vi "formas_cc.vi"(4 "retardo":dbl, 5 "Numerador":dbl[](array[numeric]), 6 "Denominador":dbl[](array[numeric])) -> (0 "Vector C":dbl[](array[numeric]), 1 "Vector B":dbl[](array[numeric]), 2 "Matriz A":T1)   [LabVIEW 2019]
doc: "Transforma una ecuacion del comportamiento del sistema( FT), a su representacion en el espacios de estados , con su numerador ,denominador y un retardo si se tiene , entregando la formas FCO."
uses:
  <vilib>/Analysis/Matrix/Datatypes/RealMatrix.ctl
  <vilib>/Analysis/7linalg.llb/Create Special Real Matrix.vi
  <vilib>/Analysis/NI_AALPro.lvlib
  <vilib>/Analysis/Matrix/NI_Matrix.lvlib
panel:
  out "Numerador 2":dbl[](array[numeric])
  out "Denominador 2":dbl[](array[numeric])
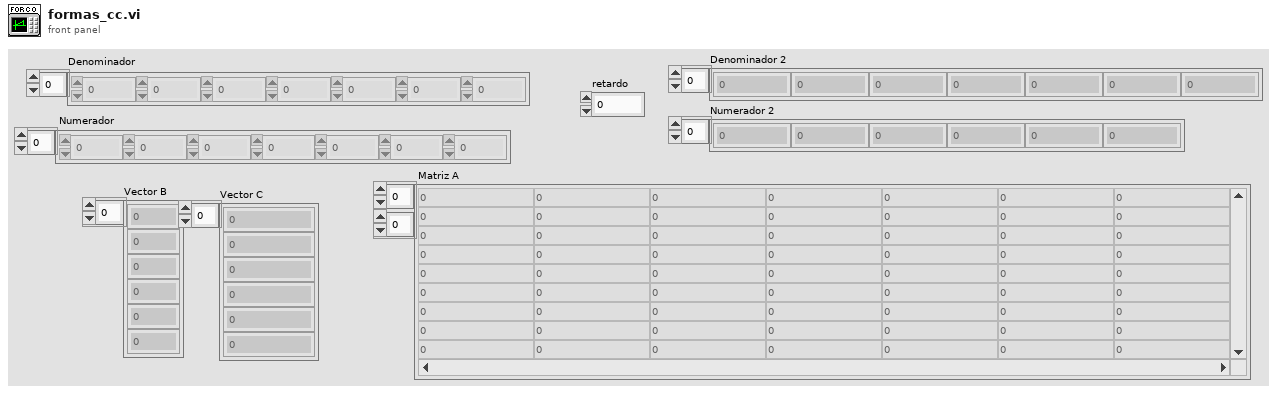
[diagram p1: front panel]
types:
  T1 = typedef "NI_Matrix.lvlib/RealMatrix.ctl" = dbl[][]
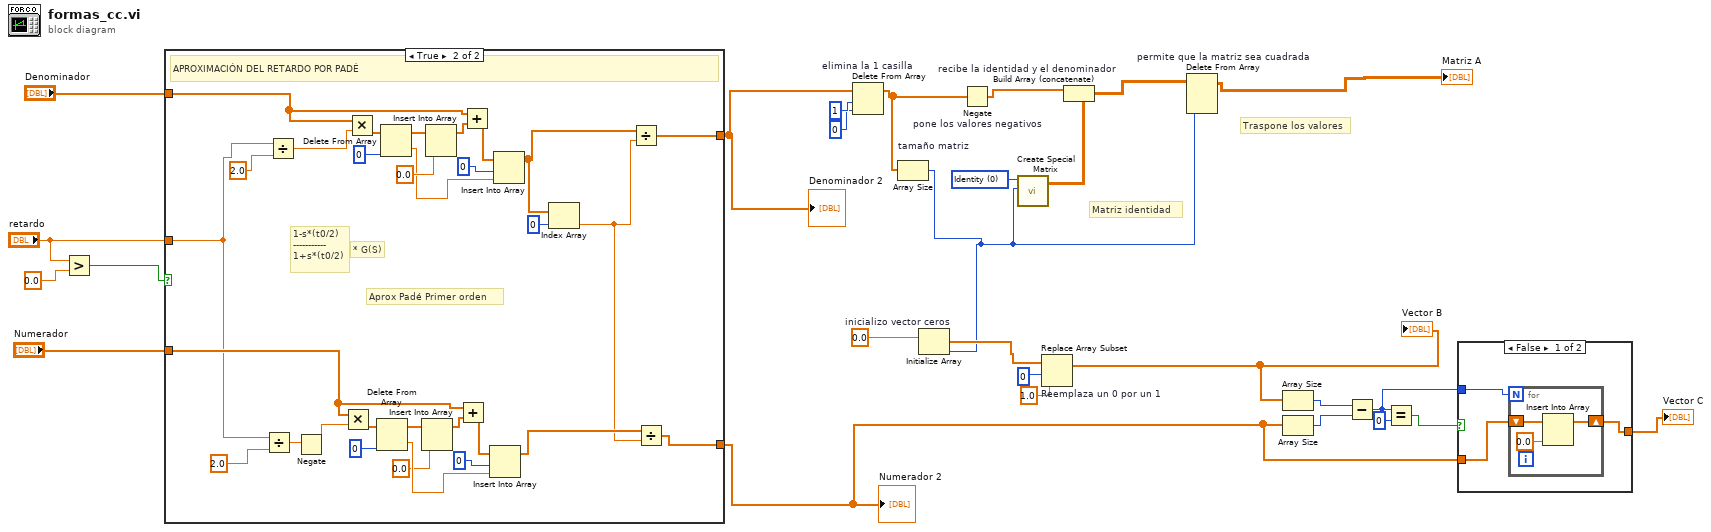
[diagram p0: block diagram]
diagram:
  w21 = 0 items=["Identity", "Diagonal", "Toeplitz", "Vandermonde", "Companion", "Hankel", "Hadamard", "Wilkinson", "Hilbert", "Inverse Hilbert", "Rosser", "Pascal"] ("matrix type")
  # "Matriz identidad"
  # "Traspone los valores"
  n1 = Greater?(x="retardo", y=0.0) -> (0:w11:bool)
  n2 = case shown="True" w11 {
    tunnel: "Numerador" -> [w28 w55]
    tunnel: "retardo" -> [_ w39]
    tunnel: "Denominador" -> [w29 w38]
    tunnel: [w28 w37] -> w3
    tunnel: [w29 w35] -> w9
    frame False {
    }
    frame True {
      # "* G(S)"
      # "Aprox Padé Primer orden"
      # "1-s*(t0/2)\n-----------\n1+s*(t0/2)"
      # "APROXIMACIÓN DEL RETARDO POR PADÉ"
      n3 = Divide(x=w39, y=2.0) -> (x/y=w36:dbl)
      n4 = Divide(x=w39, y=2.0) -> (x/y=w34:dbl)
      n5 = Negate(x=w36) -> (-x=w57:dbl)
      n6 = Multiply(x=w55, y=w57) -> (x*y=w56:dbl[])
      n7 = Multiply(x=w38, y=w34) -> (x*y=w42:dbl[])
      n8 = Delete From Array(array=w56, index=0) -> (deleted portion=w54:dbl, array with subset deleted=w52:dbl[])  [unwired: 1 in]
      n9 = Delete From Array(array=w42, index=0) -> (deleted portion=w43:dbl, array with subset deleted=w45:dbl[])  [unwired: 1 in]
      n10 = Insert Into Array(array=w52, new element=0.0 ("new element/subarray")) -> (w49:dbl[])  [unwired: 1 in]
      n11 = Insert Into Array(array=w45, new element=0.0 ("new element/subarray")) -> (w48:dbl[])  [unwired: 1 in]
      n12 = Add(x=w55, y=w49) -> (x+y=w53:dbl[])
      n13 = Add(x=w38, y=w48) -> (x+y=w44:dbl[])
      n14 = Insert Into Array(array=w53, index=0, new element=w54) -> (w31:dbl[])
      n15 = Insert Into Array(array=w44, index=0, new element=w43) -> (w33:dbl[])
      n16 = Index Array(array=w33, index=0) -> (element=w30:dbl)
      n17 = Divide(x=w33, y=w30) -> (x/y=w35:dbl[])
      n18 = Divide(x=w31, y=w30) -> (x/y=w37:dbl[])
    }
  }
  "Denominador 2" <- w9
  "Numerador 2" <- w3
  n19 = Delete From Array "elimina la 1 casilla"(array=w9, length=1, index=0) -> (array with subset deleted=w23:dbl[])  [unwired: 1 out]
  n20 = Array Size "tamaño matriz"(array=w23) -> (size(s)=w13:i32)
  n21 = Initialize Array "inicializo vector ceros"(0.0 ("element"), w13) -> (w17:dbl[])
  n22 = Negate "pone los valores negativos"(x=w23) -> (-x=w22:dbl[])
  n23 = call-poly <vilib>:"Create Special Matrix.vi"("matrix type"=w21, "matrix size"=w13) -> ("Special Matrix"=w20:T1)  [unwired: 3 in, 1 out]
  n24 = Replace Array Subset "Reemplaza un 0 por un 1"(array=w17, new element=1.0 ("new element/subarray"), index=0) -> (w8:dbl[])
  "Vector B" <- w8
  n25 = Build Array (concatenate) "recibe la identidad y el denominador"(w22, w20) -> (w19:T1)
  n26 = Delete From Array "permite que la matriz sea cuadrada"(array=w19, index (row)=w13) -> (array with subset deleted=→"Matriz A":T1)  [unwired: 2 in, 1 out]
  n27 = Array Size(array=w8) -> (size(s)=w7:i32)
  n28 = Array Size(array=w3) -> (size(s)=w6:i32)
  n29 = Subtract(x=w7, y=w6) -> (x-y=w1:i32)
  n30 = Equal?(x=w1, y=0) -> (x = y?=w4:bool)
  n31 = case shown="False" w4 {
    tunnel: w3 -> [w62 w66]
    tunnel: [w61 w66] -> w2
    tunnel: w1 -> [w60 _]
    frame False {
      n32 = for {
        N: w60 -> [_]
        shift-right: [w63] -> w61
        shift-left: w62 -> [w65]
        n33 = Insert Into Array(array=w65, new element=0.0 ("new element/subarray")) -> (w63:dbl[])  [unwired: 1 in]
      }
    }
    frame True {
    }
  }
  "Vector C" <- w2
